vi "UIRef.vi"(8 "error in":errorcluster, 11 "channel in":refnum<class "StepNode.lvclass">) -> (0 "error out":errorcluster, 2 "VI refnum":refnum<vi>, 3 "channel out":refnum<class "StepNode.lvclass">)   [LabVIEW 2015, in "StepNode.lvclass"]
doc: "Copyright 2017 National Instruments Corporation\n\nLicensed under the Apache License, Version 2.0 (the \"License\"); you may not use this file except in compliance with the License. You may obtain a copy of the License at http://www.apache.org/licenses/LICENSE-2.0\nUnless required by applicable law or agreed to in writing, software distributed under the License is distributed on an \"AS IS\" BASIS, WITHOUT WARRANTIES OR CONDITIONS OF ANY KIND, either express or implied. See the License for the specific language governing permissions and limitations under the License."
uses:
  StepNode.lvclass
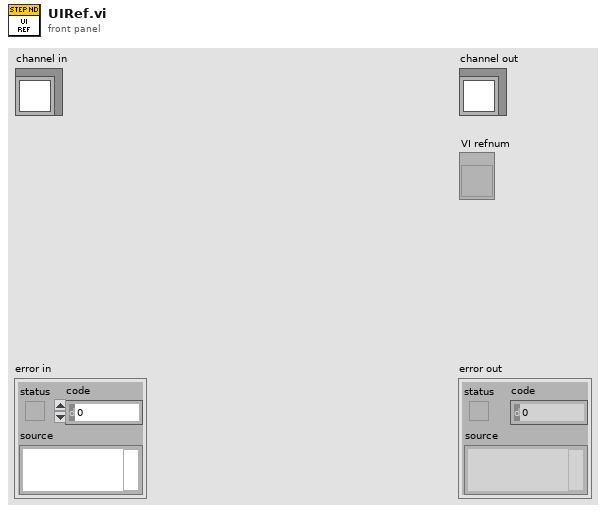
[diagram p1: front panel]
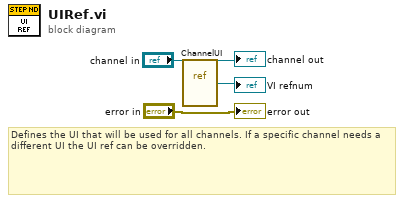
[diagram p0: block diagram]
diagram:
  # "Defines the UI that will be used for all channels. If a specific channel needs a different UI the UI ref can be overridden."
  n1 = vi-ref "ChannelUI.vi"() -> (→"VI refnum":refnum<vi>)
  "error out" <- "error in"
  "channel out" <- "channel in"
